vi "Wheel of Doom Controller.vi"(8 "error in":errorcluster) -> ()   [LabVIEW 2019]
doc: "This VI executes continuously carrying out the current operation and responding to updates or new operations. It will often contain the timing or control code that is difficult to place directly in TeleOp. This VI generally opens all sensors and motors and isolates the rest of the robot code from knowing how the operations are carried out."
uses:
  <vilib>/Rock Robotics/WPI/Framework/Completion Status.ctl
  Wheel of Doom Setpoints.ctl
  Wheel of Doom Operations.ctl
  <vilib>/Rock Robotics/WPI/ThirdParty/REV Robotics/SPARK MAX/Typedef/Spark MAX Motor Type.ctl
  <vilib>/Rock Robotics/WPI/MotorControl/WPI_MotorControlDeviceRef.ctl
  <vilib>/Rock Robotics/WPI/MotorControl/WPI_MotorControlType.ctl
  <vilib>/Rock Robotics/SystemInterfaces/DIO/FPGA_DIOPWMChannel.ctl
  <vilib>/Rock Robotics/WPI/PWM/WPI_PWMDeadband.ctl
  <vilib>/Rock Robotics/SystemInterfaces/DIO/FPGA_DIOChannel.ctl
  <vilib>/Rock Robotics/WPI/DigitalInput/WPI_DigitalInputDevRef.ctl
  <vilib>/Rock Robotics/WPI/ThirdParty/REV Robotics/Color SensorV3/Typedef/Color Sensor V3 DevRef.ctl
  <vilib>/Rock Robotics/WPI/I2C/WPI_I2CDevRef.ctl
  <vilib>/Rock Robotics/SystemInterfaces/i2clib/i2c_bus.ctl
  <vilib>/Rock Robotics/WPI/Interrupt/WPI_InterruptRef.ctl
  <vilib>/Rock Robotics/SystemInterfaces/Interrupt/FPGA_InterruptIndex.ctl
  Wheel of Doom Slot State.ctl
  <vilib>/Rock Robotics/WPI/ThirdParty/REV Robotics/Color SensorV3/Typedef/Color Sensor V3 ProximityRate.ctl
  <vilib>/Rock Robotics/WPI/ThirdParty/REV Robotics/Color SensorV3/Typedef/Color Sensor V3 ProxResolution.ctl
  <vilib>/Rock Robotics/WPI/Counter/WPI_CounterDevRef.ctl
  <vilib>/Rock Robotics/SystemInterfaces/Counter/FPGA_CounterCtrSystemIndex.ctl
  <vilib>/Rock Robotics/WPI/ThirdParty/REV Robotics/SPARK MAX/Typedef/Spark MAX Status Frames.ctl
  <vilib>/Rock Robotics/WPI/ThirdParty/REV Robotics/SPARK MAX/Typedef/Spark MAX Control Type.ctl
  <vilib>/Rock Robotics/WPI/Counter/WPI_CounterDigitalInputToDigitalSource.vi
  <vilib>/Rock Robotics/SystemInterfaces/CounterEncoderSourceConvertion/FPGA_CounterEncoderSourceConvertionLVSourceTypeToFPGAType.vi
  <vilib>/Rock Robotics/WPI/Interrupt/WPI_InterruptCache.vi
  <vilib>/Rock Robotics/SystemInterfaces/Interrupt/FPGA_InterruptWriteConfiguration.vi
  Wheel of Doom State.vi
  Wheel of Doom Internal Global.vi
  <vilib>/Rock Robotics/SystemInterfaces/Interrupt/FPGA_WaitOnInterrupt.vi
  <vilib>/Rock Robotics/WPI/Utilities/WPI_UtilitiesTimebaseConstants.vi
  <vilib>/Rock Robotics/SystemInterfaces/Interrupt/FPGA_InterruptReadTimestamp.vi
  <vilib>/ptbypt/NI_PtbyPt.lvlib
panel:
  in  "Auto-Karen Speed":dbl=0.19
  in  "Reverse Time":u32=600
  out "Current Trip":bool
  in  "Intake Mode Current Trigger":dbl=15.0
  in  "Intake Mode Speed":dbl=0.19
  out "Shoot All Complete":bool=TRUE
  in  "Shoot All Time (ms)":u32=3000
  in  "Wheel of Doom Shot Voltage":dbl=4.4
  out "Current Slot":u32=4
  out "State":cluster{"Valid":bool, "State":bool}[](array[cluster])=[{"Valid"=FALSE, "State"=FALSE}, {"Valid"=FALSE, "State"=FALSE}, {"Valid"=FALSE, "State"=FALSE}, {"Valid"=FALSE, "State"=FALSE}, {"Valid"=TRUE, "State"=FALSE}, {"Valid"=FALSE, "State"=FALSE}]
  out "Sensor Data":cluster{"Prox Threshold":u16, dbl}(graph)={"Prox Threshold"=14, 341.057373046875}
  in  "Prox Threshold":u16=30
  in  "Sensor Sample Start Pos":dbl
  in  "Sensor Sample End Pos":dbl
  in  "Interactive Values":T1
  out "Current\nCmd":string="Started at  19:17:32.261\n: Immediate,  S 0.0, D 0.000000"
  in  "Buttons":cluster{"Execute Cmd":bool, "Abort Cmd":bool}
  out "Command Timing":cluster{"Start Time (ms)":u32, "Iterations":i32}={"Start Time (ms)"=527443, "Iterations"=0}
  out "Status":T3
  # "Interactive Command: You may fill in the settings for a command\nand schedule it with the Execute button. You can observe and abort\nany command while fine tuning the code for the controller."
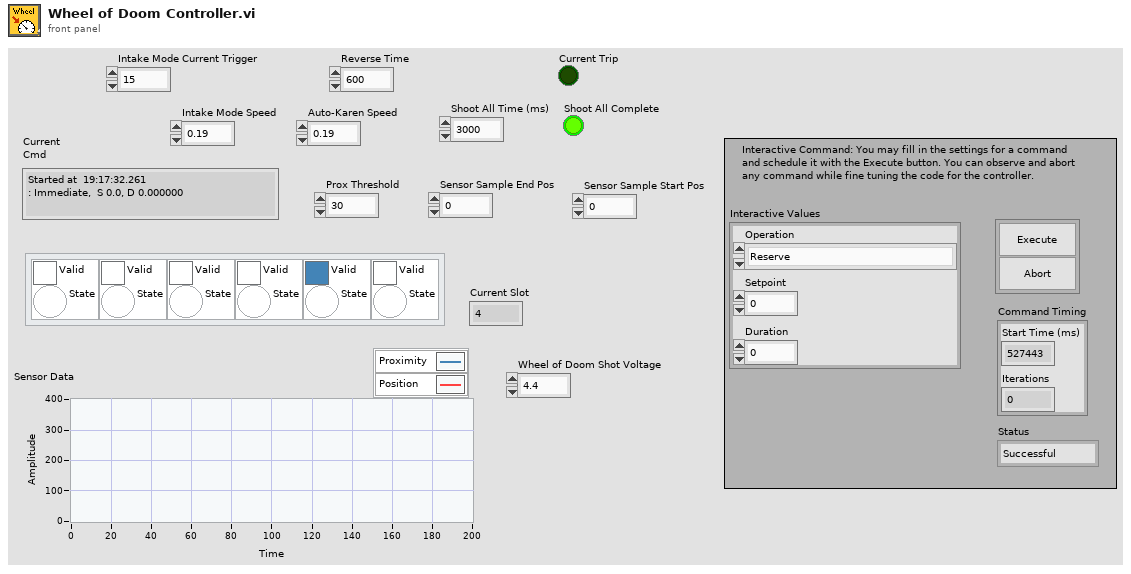
[diagram p1: front panel]
types:
  T1 = typedef "Wheel of Doom Setpoints.ctl" = cluster{"Operation":T2, "Setpoint":dbl, "Duration":dbl}
  T2 = typedef "Wheel of Doom Operations.ctl" = enum16{"Reserve", "Read Current", "Immediate", "Intake Mode", "Stop on Empty", "Shoot All", "Shoot One", "Stop", "Auto Karen"}
  T3 = typedef "Completion Status.ctl" = enum16{"Successful", "Aborted", "Incomplete"}
  T4 = typedef "Spark MAX Status Frames.ctl" = enum16{"Status 0", "Status 1", "Status 2", "Status 3"}
  T5 = typedef "Wheel of Doom Slot State.ctl" = cluster{"Slot Seen?":bool, "Ball Present":bool}
  T6 = typedef "WPI_MotorControlDeviceRef.ctl" = cluster{"DeviceStatus":errorcluster, "Type":T7, "PWM":cluster{"PWM Channel":T8, "DeadBand":T9}, "CAN":cluster{"Device Number":u8, "SetOutput VI Ref":variant, "GetOutput VI Ref":variant, "Enable VI Ref":variant, "Disable VI Ref":variant, "Data":variant}, "Invert":bool, "DIO PWM":cluster{"PWM \"Enable\" Channel":T8, "DIOChannel":T10, "PWM Rate":dbl}}
  T7 = typedef "WPI_MotorControlType.ctl" = enum16{"PWM", "CAN", "DIO PWM"}
  T8 = typedef "FPGA_DIOPWMChannel.ctl" = enum8{"PWM 0", "PWM 1", "PWM 2", "PWM 3", "PWM 4", "PWM 5", "PWM 6", "PWM 7", "PWM 8", "PWM 9", "PWM MXP 0", "PWM MXP 1", "PWM MXP 2", "PWM MXP 3", "PWM MXP 4", "PWM MXP 5", "PWM MXP 6", "PWM MXP 7", "PWM MXP 8", "PWM MXP 9", "Invalid"}
  T9 = typedef "WPI_PWMDeadband.ctl" = cluster{"Name":string, "maxPositivePwm":i32, "minPositivePwm":i32, "centerPwm":i32, "maxNegativePwm":i32, "minNegativePwm":i32, "angularRange":u16}
  T10 = typedef "FPGA_DIOChannel.ctl" = enum8{"DIO 0", "DIO 1", "DIO 2", "DIO 3", "DIO 4", "DIO 5", "DIO 6", "DIO 7", "DIO 8", "DIO 9", "DIO MXP 0", "DIO MXP 1", "DIO MXP 2", "DIO MXP 3", "DIO MXP 4", "DIO MXP 5", "DIO MXP 6", "DIO MXP 7", "DIO MXP 8", "DIO MXP 9", "DIO MXP 10", "DIO MXP 11", "DIO MXP 12", "DIO MXP 13", "DIO MXP 14", "DIO MXP 15", "SPI Port CS1", "SPI Port CS2", "SPI Port CS3", "SPI Port MISO", "SPI Port MOSI", "Invalid"}
  T11 = typedef "WPI_CounterDevRef.ctl" = cluster{"DevStatus":errorcluster, "CntIndex":T12}
  T12 = typedef "FPGA_CounterCtrSystemIndex.ctl" = enum8{"Ctr 0", "Ctr 1", "Ctr 2", "Ctr 3", "Ctr 4", "Ctr 5", "Ctr 6", "Ctr 7", "Invalid"}
  T13 = typedef "i2c_bus.ctl" = enum16{"I2C On-Board", "I2C MXP", "Invalid"}
  T14 = typedef "Color Sensor V3 ProxResolution.ctl" = enum8{"8bit", "9bit", "10bit", "11bit"}
  T15 = typedef "Color Sensor V3 ProximityRate.ctl" = enum16{"6ms", "12ms", "25ms", "50ms", "100ms", "200ms", "400ms"}
  T16 = typedef "WPI_DigitalInputDevRef.ctl" = cluster{"DevStatus":errorcluster, "DIO Channel":T10}
  T17 = typedef "Color Sensor V3 DevRef.ctl" = cluster{"I2CDevRef":T18}
  T18 = typedef "WPI_I2CDevRef.ctl" = cluster{"DevStatus":errorcluster, "Device Address":u8, "Handle":i32, "I2C Bus":T13}
  T19 = typedef "WPI_InterruptRef.ctl" = cluster{"DevStatus":errorcluster, "InterruptIndex":T20}
  T20 = typedef "FPGA_InterruptIndex.ctl" = enum8{"0", "1", "2", "3", "4", "5", "6", "7", "Invalid"}
  T21 = cluster{"Motor":T6, "Mag Switch":T16, "Prox Sensor":T17, "Interrupt":T19, "Slot States":T5[]}
  T22 = typedef "Spark MAX Motor Type.ctl" = enum16{"Brushed", "Brushless"}
  T23 = typedef "FPGA_CounterEncoderSourceConvertionLVSourceType.ctl" = cluster{"DevStatus":errorcluster, "AnalogTriggerMode?":bool, "DigitalMode":cluster{"DIO Channel":T24}, "AnalogTriggerMode":cluster{"AnalogTriggerIndex":T25, "OutputType":T26}}
  T24 = typedef "FPGA_DIODigitalSourceChannel.ctl" = enum8{"DIO 0", "DIO 1", "DIO 2", "DIO 3", "DIO 4", "DIO 5", "DIO 6", "DIO 7", "DIO 8", "DIO 9", "DIO MXP 0", "DIO MXP 1", "DIO MXP 2", "DIO MXP 3", "DIO MXP 4", "DIO MXP 5", "DIO MXP 6", "DIO MXP 7", "DIO MXP 8", "DIO MXP 9", "DIO MXP 10", "DIO MXP 11", "DIO MXP 12", "DIO MXP 13", "DIO MXP 14", "DIO MXP 15", "SPI Port CS1", "SPI Port CS2", "SPI Port CS3", "SPI Port MISO", "SPI Port MOSI", "Disabled"}
  T25 = typedef "FPGA_AnalogTriggerIndex.ctl" = enum8{"Trig 0", "Trig 1", "Trig 2", "Trig 3", "Trig 4", "Trig 5", "Trig 6", "Trig 7", "Invalid"}
  T26 = typedef "FPGA_AnalogTriggerOutType.ctl" = enum16{"InWindow", "TriggerState", "Rising", "Falling"}
  T27 = typedef "Command Status Info.ctl" = cluster{"Name":string, "Status":T3, "notifier out":T28}
  T28 = typedef "Completion Notifier.ctl" = refnum<notifier>
  T29 = cluster{"Current Command":T1, "Command Timing":cluster{"Start Time (ms)":u32, "Iterations":i32}, "Command Arguments":cluster{"Command Info":T27, "Description":string, "Default Command":T1, "queue out":refnum<queue>, "Subsystem Name":string}}
  T30 = typedef "Spark MAX Control Type.ctl" = enum16{"Percent VBus", "Voltage", "Velocity", "Position", "Smart Motion", "Current", "Smart Velocity"}
  T31 = cluster{"Proximity":u16, "Normalized Sensor Positon":dbl}
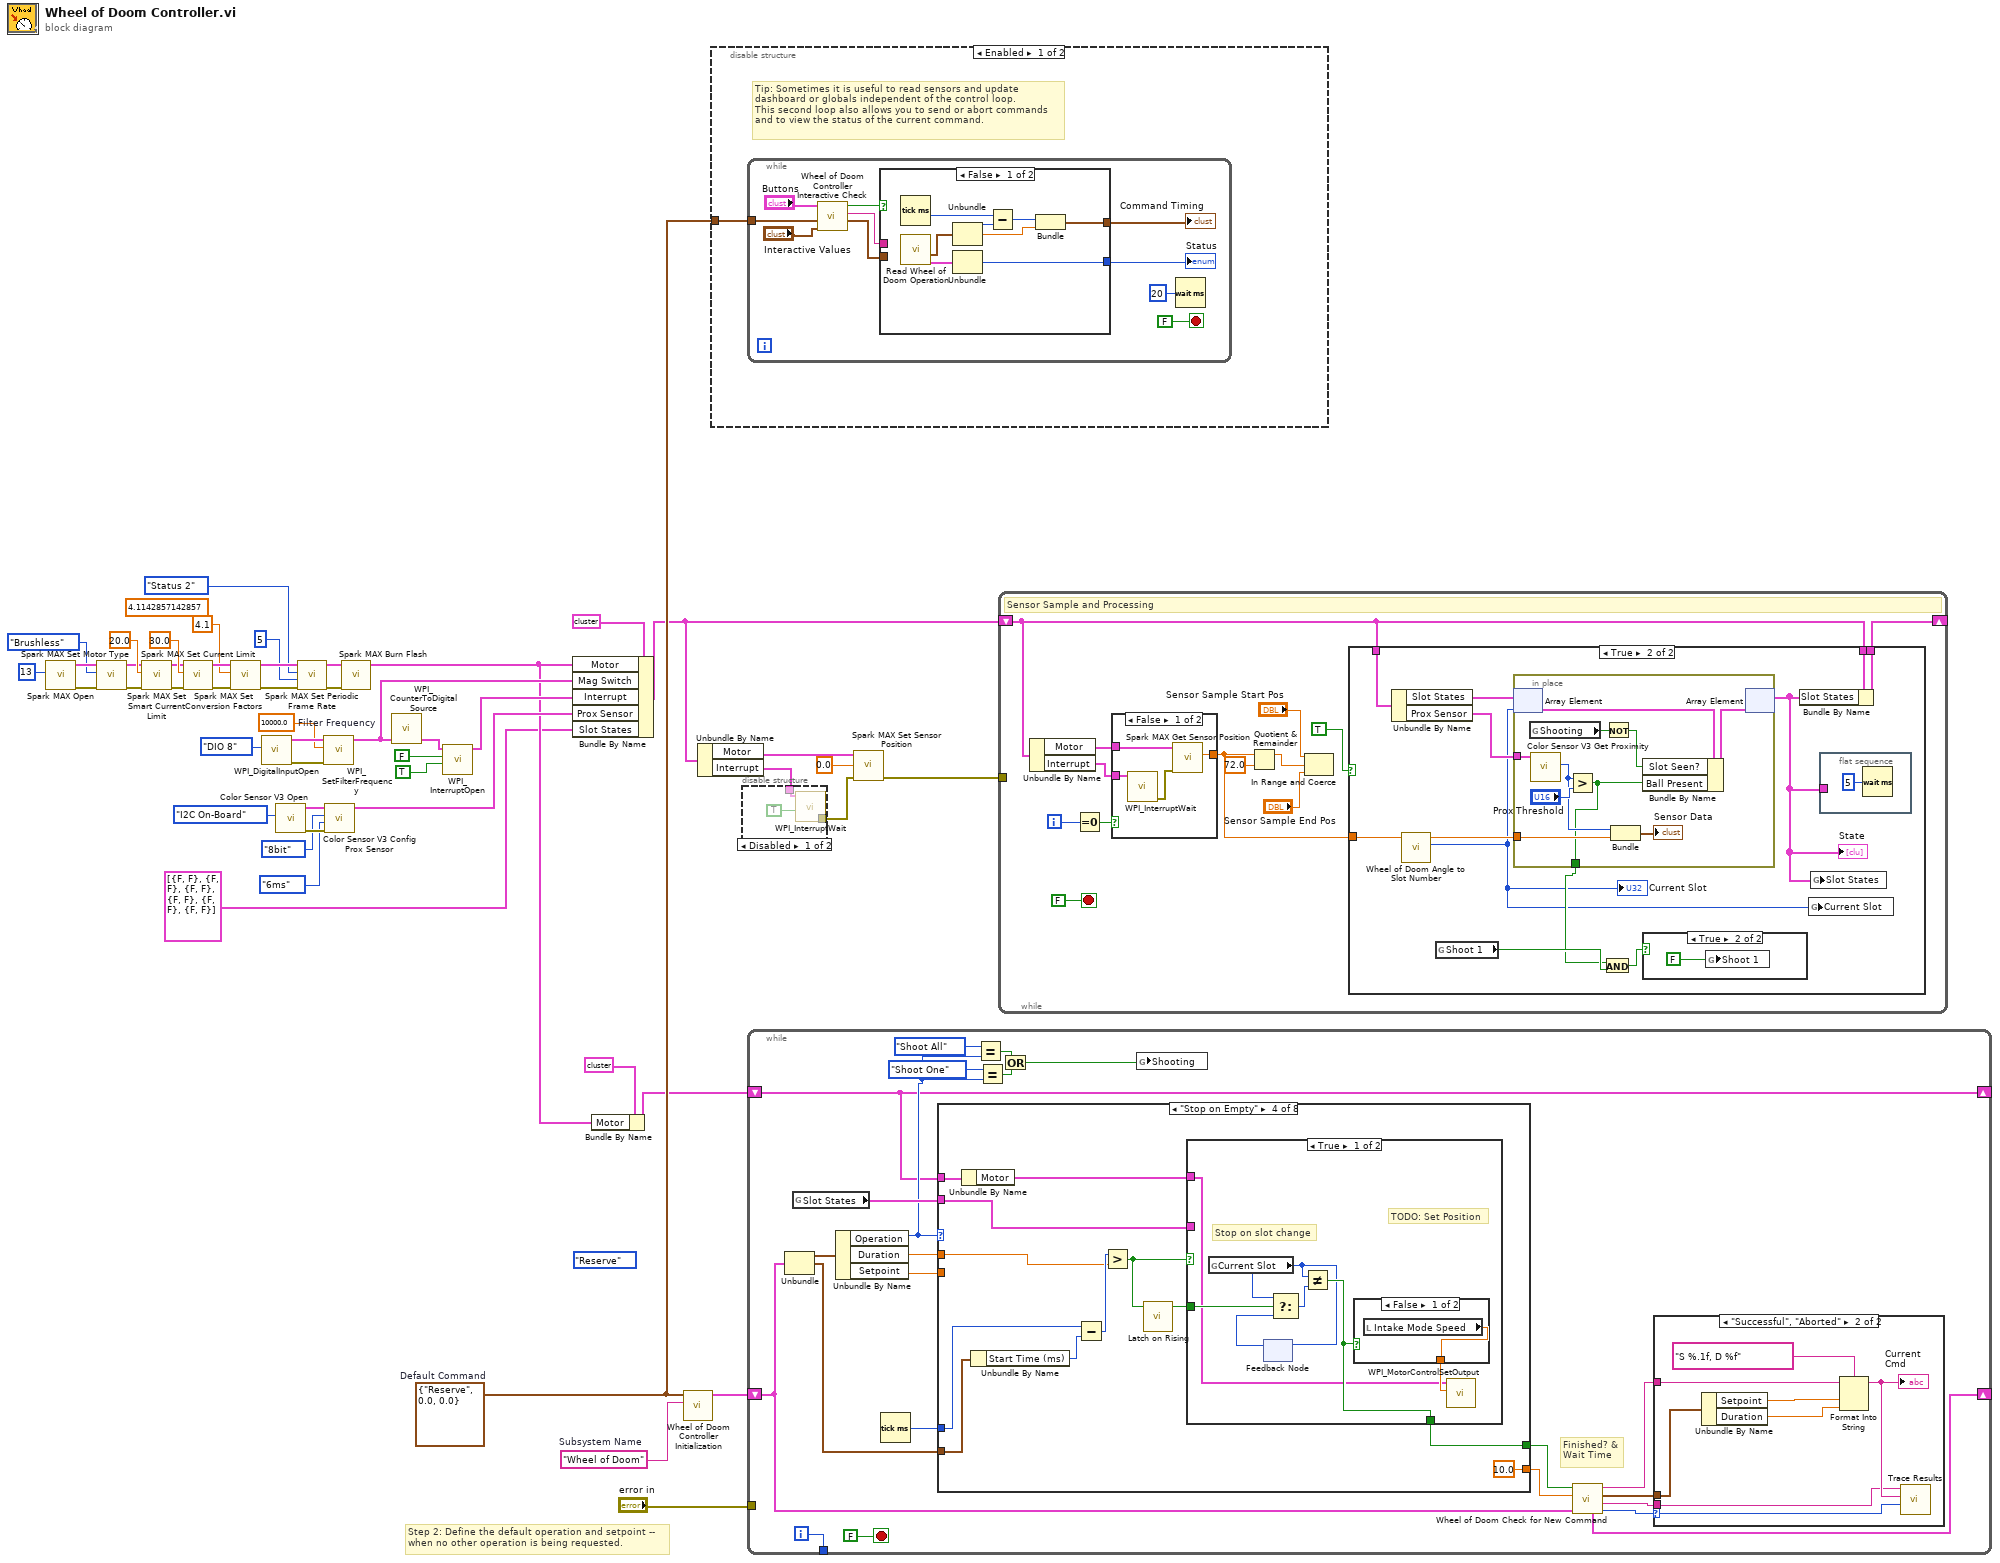
[diagram p0: block diagram]
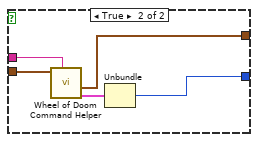
[diagram p2: hidden frame]
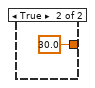
[diagram p5: hidden frame]
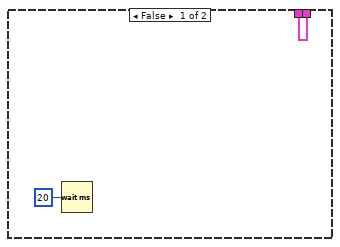
[diagram p6: hidden frame]
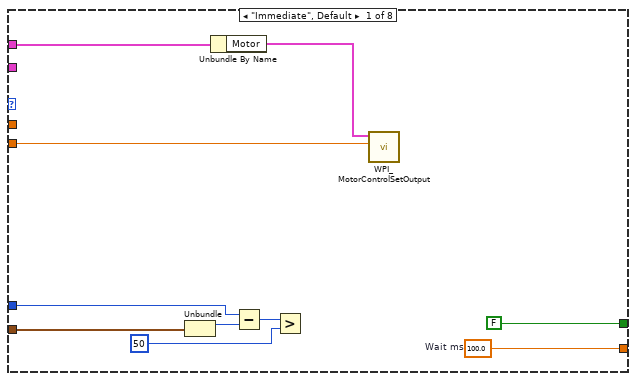
[diagram p9: hidden frame]
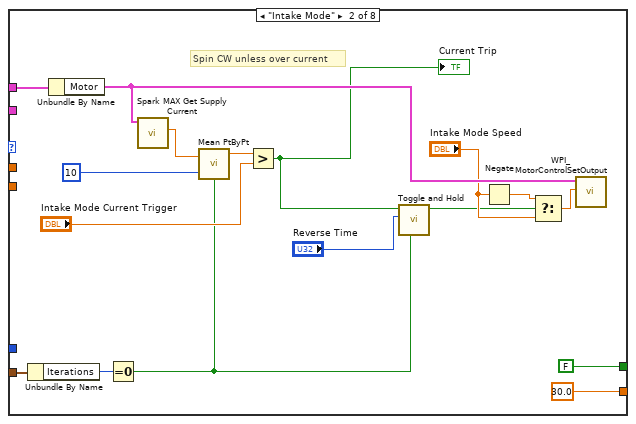
[diagram p10: hidden frame]
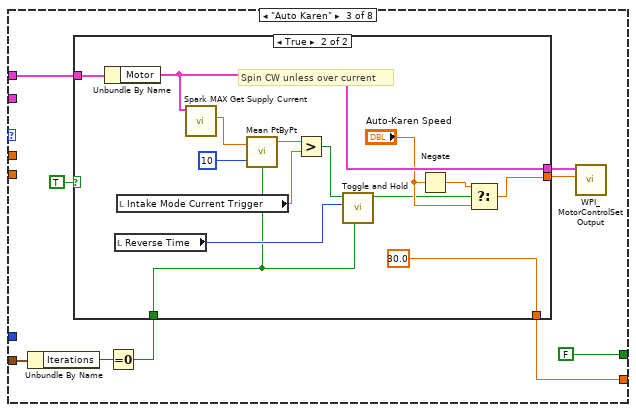
[diagram p11: hidden frame]
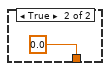
[diagram p13: hidden frame]
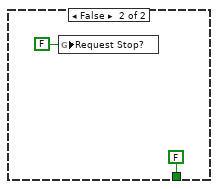
[diagram p14: hidden frame]
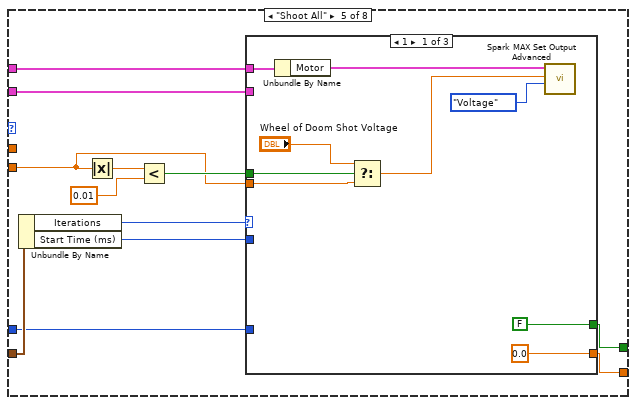
[diagram p15: hidden frame]
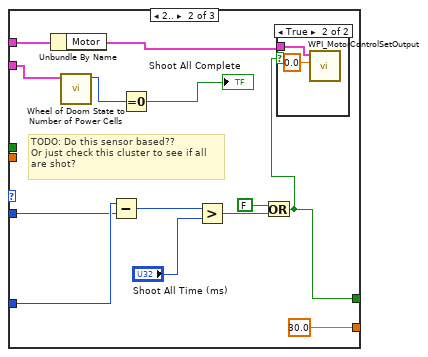
[diagram p16: hidden frame]
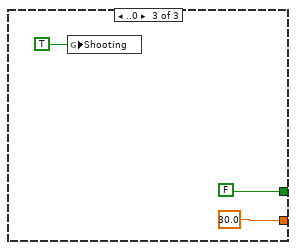
[diagram p18: hidden frame]
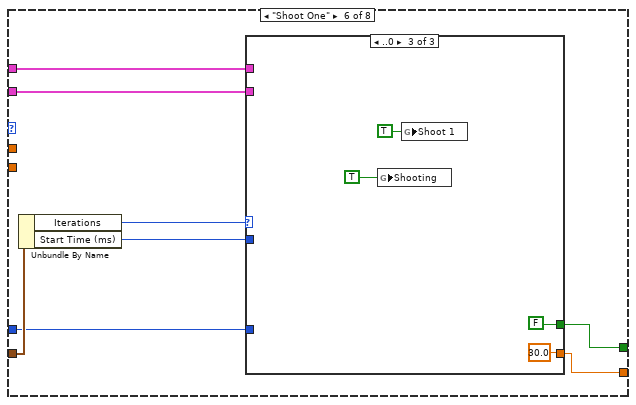
[diagram p19: hidden frame]
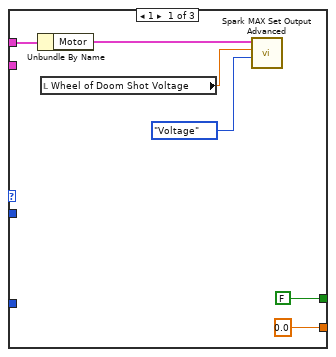
[diagram p20: hidden frame]
diagram:
  (unwired) 4.1142857142857 ("Position Factor (1)")
  (unwired) Wheel_of_Doom_Operations."Reserve" ("Operation")
  w31 = 10000.0  # Filter Frequency
  w46 = T1 {"Operation"=enum."Reserve", "Setpoint"=0.0, "Duration"=0.0}  # Default Command
  w47 = "Wheel of Doom"  # Subsystem Name
  # "Step 2: Define the default operation and setpoint --\nwhen no other operation is being requested."
  n1 = call <vilib>:"Spark MAX Open.vi"("Device Number"=u8 13) -> ("error out"=w42:errorcluster, "MotorControlDeviceRef"=w38:T6)  [unwired: 9 in]
  n2 = call <vilib>:"Spark MAX Set Motor Type.vi"("error in (no error)"=w42, "Motor Type"=Spark_MAX_Motor_Type."Brushless", "MotorControlDevRef"=w38) -> ("error out"=w39:errorcluster, "MotorControlDeviceRef"=w37:T6)  [unwired: 7 in]
  n3 = call <vilib>:"Spark MAX Set Smart Current Limit.vi"("error in (no error)"=w39, "Primay Current Limit (80A)"=20.0, "MotorControlDeviceRef in"=w37) -> ("error out"=w40:errorcluster, "MotorControlDeviceRef out"=w41:T6)  [unwired: 7 in]
  n4 = call <vilib>:"Spark MAX Set Current Limit.vi"("error in (no error)"=w40, "Current Limit A (100)"=sgl 30.0, "MotorControlDeviceRef in"=w41) -> ("error out"=w35:errorcluster, "MotorControlDeviceRef out"=w8:T6)  [unwired: 7 in]
  n5 = call <vilib>:"Spark MAX Set Conversion Factors.vi"("error in (no error)"=w35, "Position Factor (1)"=4.1, "MotorControlDeviceRef in"=w8) -> ("error out"=w9:errorcluster, "MotorControlDeviceRef out"=w6:T6)  [unwired: 7 in]
  n6 = call <vilib>:"WPI_DigitalInputOpen.vi"("DIO Channel"=FPGA_DIOChannel."DIO 8") -> ("error out"=w32:errorcluster, "DigitalInputDevRef"=w34:T16)  [unwired: 9 in]
  n7 = call <vilib>:"Color Sensor V3 Open.vi"("I2C Bus"=i2c_bus."I2C On-Board") -> ("error out"=w30:errorcluster, "ColorSensorDevRef"=w29:T17)  [unwired: 9 in]
  n8 = call <vilib>:"Spark MAX Set Periodic Frame Rate.vi"("error in"=w9, "Frame rate (ms)"=u16 5, "Frame"=Spark_MAX_Status_Frames."Status 2", "MotorControlDeviceRef"=w6) -> ("error out"=w7:errorcluster, "MotorControlDeviceRef"=w5:T6)  [unwired: 6 in]
  n9 = call <vilib>:"WPI_SetFilterFrequency.vi"("error in (no error)"=w32, "Filter Frequency"=w31, "DigitalInputDevRef"=w34) -> ("DigitalInputDevRef"=w25:T16)  [unwired: 7 in, 1 out]
  n10 = call <vilib>:"Color Sensor V3 Config Prox Sensor.vi"("error in (no error)"=w30, "ProximitySensorMeasurementRate"=Color_Sensor_V3_ProximityRate."6ms", "ProximitySensorResolution"=Color_Sensor_V3_ProxResolution."8bit", "ColorSensorDevRef"=w29) -> ("ColorSensorDevRef out"=w17:T17)  [unwired: 6 in, 1 out]
  n11 = call <vilib>:"Spark MAX Burn Flash.vi"("error in"=w7, "MotorControlDeviceRef"=w5) -> ("MotorControlDeviceRef"=w11:T6)  [unwired: 8 in, 1 out]
  n12 = call-poly <vilib>:"WPI_CounterToDigitalSource.vi"("DigitalInputDevRef"=w25) -> ("Digital Source"=w24:T23)  [unwired: 6 in]
  n13 = call <vilib>:"WPI_InterruptOpen.vi"("Falling Edge"=TRUE, "Rising Edge"=FALSE, "Source"=w24) -> ("InterruptRef"=w16:T19)  [unwired: 7 in, 1 out]
  n14 = Bundle By Name(cluster=T21 {"Motor"={"DeviceStatus"={"status"=FALSE, "code"=0, "source"=""}, "Type"=enum."PWM", "PWM"={"PWM Channel"=enum."Invalid", "DeadBand"={"Name"="", "maxPositivePwm"=0, "minPositivePwm"=0, "centerPwm"=0, "maxNegativePwm"=0, "minNegativePwm"=0, "angularRange"=0}}, "CAN"={"Device Number"=0, "SetOutput VI Ref"=variant(refnum<vi> refnum), "GetOutput VI Ref"=variant(refnum<vi> refnum), "Enable VI Ref"=variant(refnum<vi> refnum), "Disable VI Ref"=variant(refnum<vi> refnum), "Data"=variant}, "Invert"=FALSE, "DIO PWM"={"PWM \"Enable\" Channel"=enum."Invalid", "DIOChannel"=enum."Invalid", "PWM Rate"=0.0}}, "Mag Switch"={"DevStatus"={"status"=FALSE, "code"=0, "source"=""}, "DIO Channel"=enum."DIO 1"}, "Prox Sensor"={"I2CDevRef"={"DevStatus"={"status"=FALSE, "code"=0, "source"=""}, "Device Address"=0, "Handle"=0, "I2C Bus"=enum."Invalid"}}, "Interrupt"={"DevStatus"={"status"=FALSE, "code"=0, "source"=""}, "InterruptIndex"=enum."Invalid"}, "Slot States"=[{"Slot Seen?"=FALSE, "Ball Present"=FALSE}, {"Slot Seen?"=FALSE, "Ball Present"=FALSE}, {"Slot Seen?"=FALSE, "Ball Present"=FALSE}, {"Slot Seen?"=FALSE, "Ball Present"=FALSE}, {"Slot Seen?"=FALSE, "Ball Present"=FALSE}]}, "Motor"=w11, "Mag Switch"=w25, "Interrupt"=w16, "Prox Sensor"=w17, "Slot States"=T5[] [{"Slot Seen?"=FALSE, "Ball Present"=FALSE}, {"Slot Seen?"=FALSE, "Ball Present"=FALSE}, {"Slot Seen?"=FALSE, "Ball Present"=FALSE}, {"Slot Seen?"=FALSE, "Ball Present"=FALSE}, {"Slot Seen?"=FALSE, "Ball Present"=FALSE}, {"Slot Seen?"=FALSE, "Ball Present"=FALSE}]) -> (w2:T21)
  n15 = Bundle By Name(cluster=cluster{"Motor":T6, "Ball Detect2":T11} {"Motor"={"DeviceStatus"={"status"=FALSE, "code"=0, "source"=""}, "Type"=enum."PWM", "PWM"={"PWM Channel"=enum."Invalid", "DeadBand"={"Name"="", "maxPositivePwm"=0, "minPositivePwm"=0, "centerPwm"=0, "maxNegativePwm"=0, "minNegativePwm"=0, "angularRange"=0}}, "CAN"={"Device Number"=0, "SetOutput VI Ref"=variant(refnum<vi> refnum), "GetOutput VI Ref"=variant(refnum<vi> refnum), "Enable VI Ref"=variant(refnum<vi> refnum), "Disable VI Ref"=variant(refnum<vi> refnum), "Data"=variant}, "Invert"=FALSE, "DIO PWM"={"PWM \"Enable\" Channel"=enum."Invalid", "DIOChannel"=enum."Invalid", "PWM Rate"=0.0}}, "Ball Detect2"={"DevStatus"={"status"=FALSE, "code"=0, "source"=""}, "CntIndex"=enum."Ctr 0"}}, "Motor"=w11) -> (w12:cluster{"Motor":T6, "Ball Detect2":T11})
  n16 = call "Wheel of Doom Controller Initialization.vi"("Subsystem Name"=w47, "Default Command"=w46) -> ("Current Command"=w48:T29)  [unwired: 9 in]
  n17 = Unbundle By Name(w2) -> ("Motor"=w20:T6, "Interrupt"=w14:T19)
  n18 = disable-structure shown="Enabled" {
    disable-tunnel: w46 -> [w50 _]
    frame Enabled {
      # "Tip: Sometimes it is useful to read sensors and update\ndashboard or globals independent of the control loop.\nThis second loop also allows you to send or abort commands\nand to view the status of the current command."
      n19 = while {
        tunnel: w50 -> [w57]
        stop <- FALSE stop-if-true
        n20 = call "Wheel of Doom Controller Interactive Check.vi"("Interactive Command in"="Interactive Values", "Default Command"=w57, "Buttons"="Buttons") -> ("Interactive Command out"=w54:T1, "Trace String"=w55:string, "Schedule"=w56:bool)  [unwired: 6 in]
        n21 = case shown="False" w56 {
          tunnel: [w68 w73] -> w53
          tunnel: w54 -> [_ w71]
          tunnel: [w64 w69] -> w52
          tunnel: w55 -> [_ w72]
          frame False {
            n22 = Tick Count (ms)() -> (millisecond timer value=w63:u32)
            n23 = call "Read Wheel of Doom Operation.vi"() -> ("Command Info"=w61:T27, "SubSystem Data"=w62:T1)  [unwired: 9 in, 1 out]
            n24 = Unbundle(w62) -> ("Operation"=w67:T2, "Setpoint"=w65:dbl)  [unwired: 1 out]
            n25 = Unbundle(w61) -> ("Status"=w68:T3)  [unwired: 2 out]
            n26 = Subtract(x=w63, y=w67) -> (x-y=w66:u32)
            n27 = Bundle(w66, "Setpoint"=w65) -> (w64:cluster{u32, "Setpoint":dbl})  [unwired: 1 in]
          }
          frame True {
            n28 = call "Wheel of Doom Command Helper.vi"("Description"=w72, "SubSystem Data"=w71) -> ("Command Info Out"=w70:T27, "Command Timing"=w69:cluster{"Start Time (ms)":u32, "Iterations":i32})  [unwired: 7 in, 1 out]
            n29 = Unbundle(w70) -> ("Status"=w73:T3)  [unwired: 2 out]
          }
        }
        "Status" <- w53
        "Command Timing" <- w52
        n30 = Wait (ms)(milliseconds to wait=u32 20) -> ()  [unwired: 1 out]
      }
    }
    frame Disabled {
    }
  }
  n31 = disable-structure shown="Disabled" {
    disable-tunnel: [w75 _] -> w21
    disable-tunnel: w14 -> [w74 _]
    frame Disabled {
      n32 = call <vilib>:"WPI_InterruptWait.vi"("Ignore Previous Interrupts"=TRUE, "InterruptRef"=w74) -> ("error out"=w75:errorcluster)  [unwired: 5 in, 4 out]
    }
    frame Enabled {
    }
  }
  n33 = while {
    shift-right: [w93] -> _
    shift-left: w48 -> [w86]
    tunnel: [w98] -> _
    tunnel: "error in" -> [_]
    shift-right: [w77] -> _
    shift-left: w12 -> [w77]
    i -> [w98]
    stop <- FALSE stop-if-true
    # "Finished? &\nWait Time"
    n34 = Unbundle(w86) -> ("Current Command"=w97:T1, "Command Timing"=w95:cluster{"Start Time (ms)":u32, "Iterations":i32})  [unwired: 1 out]
    n35 = global read "Wheel of Doom State.vi" "Slot States"() -> (w84:T5[])
    n36 = Unbundle By Name(w97) -> ("Operation"=w80:T2, "Duration"=w85:dbl, "Setpoint"=w94:dbl)
    n37 = Tick Count (ms)() -> (millisecond timer value=w96:u32)
    n38 = case shown="\"Stop on Empty\"" w80 {
      tunnel: [w117 30.0 ("Infinite") w142 10.0 ("Infinite") w189 w224 w246 0.0 ("Infinite")] -> w91
      tunnel: [FALSE ("ignore previous (F)") FALSE ("ignore previous (F)") FALSE ("ignore previous (F)") w165 w188 w223 FALSE ("ignore previous (F)") TRUE ("ignore previous (F)")] -> w92
      tunnel: w95 -> [w113 w130 w139 w166 w192 w227 _ _]
      tunnel: w85 -> [_ _ _ w160 _ _ _ _]
      tunnel: w96 -> [w112 _ _ w162 w187 w222 _ _]
      tunnel: w94 -> [w109 _ _ _ w181 _ _ _]
      tunnel: w84 -> [_ _ _ w167 w185 w220 _ _]
      tunnel: w77 -> [w111 w132 w141 w169 w190 w225 _ w249]
      frame "Immediate", Default {
        w117 = 100.0  # Wait ms
        n39 = Unbundle(w113) -> ("Start Time (ms)"=w116:u32)  [unwired: 1 out]
        n40 = Unbundle By Name(w111) -> ("Motor"=w110:T6)
        n41 = Subtract(x=w112, y=w116) -> (x-y=w115:u32)
        n42 = Greater?(x=w115, y=u8 50 ("Left Motor")) -> ()  [unwired: 1 out]
        n43 = call <vilib>:"WPI_MotorControlSetOutput.vi"("Output"=w109, "MotorControlDevRef"=w110) -> ()  [unwired: 7 in, 3 out]
      }
      frame "Intake Mode" {
        # "Spin CW unless over current"
        n44 = Unbundle By Name(w130) -> ("Iterations"=w129:i32)
        n45 = Unbundle By Name(w132) -> ("Motor"=w131:T6)
        n46 = Equal To 0?(x=w129) -> (x = 0?=w120:bool)
        n47 = call <vilib>:"Spark MAX Get Supply Current.vi"("MotorControlDevRef in"=w131) -> ("Current"=w127:dbl)  [unwired: 7 in, 3 out]
        n48 = call <vilib>:"Mean PtByPt.vi"("x"=w127, "sample length"=10, "initialize"=w120) -> ("mean"=w126:dbl)  [unwired: 1 in, 1 out]
        n49 = Greater?(x=w126, y="Intake Mode Current Trigger") -> (0:w118:bool)
        "Current Trip" <- w118
        n50 = call "Toggle and Hold.vi"("Reset? (F)"=w120, "Hold Time (ms)"="Reverse Time", "Trigger"=w118) -> ("Toggled?"=w119:bool)  [unwired: 7 in, 1 out]
        n51 = Negate(x="Intake Mode Speed") -> (-x=w123:dbl)
        n52 = Select(t=w123, s=w119, f="Intake Mode Speed") -> (s? t:f=w124:dbl)
        n53 = call <vilib>:"WPI_MotorControlSetOutput.vi"("Output"=w124, "MotorControlDevRef"=w131) -> ()  [unwired: 7 in, 3 out]
      }
      frame "Auto Karen" {
        n54 = Unbundle By Name(w139) -> ("Iterations"=w138:i32)
        n55 = Equal To 0?(x=w138) -> (x = 0?=w137:bool)
        n56 = case shown="True" TRUE {
          tunnel: [_ 30.0 ("Infinite")] -> w142
          tunnel: w141 -> [_ w156]
          tunnel: [_ w155] -> w140
          tunnel: w137 -> [_ w146]
          tunnel: [_ w144] -> w136
          frame False {
          }
          frame True {
            # "Spin CW unless over current"
            n57 = Unbundle By Name(w156) -> ("Motor"=w155:T6)
            n58 = local read "Reverse Time"() -> (w147:u32)
            n59 = local read "Intake Mode Current Trigger"() -> (w148:dbl)
            n60 = call <vilib>:"Spark MAX Get Supply Current.vi"("MotorControlDevRef in"=w155) -> ("Current"=w153:dbl)  [unwired: 7 in, 3 out]
            n61 = call <vilib>:"Mean PtByPt.vi"("x"=w153, "sample length"=10, "initialize"=w146) -> ("mean"=w152:dbl)  [unwired: 1 in, 1 out]
            n62 = Greater?(x=w152, y=w148) -> (0:w145:bool)
            n63 = call "Toggle and Hold.vi"("Reset? (F)"=w146, "Hold Time (ms)"=w147, "Trigger"=w145) -> ("Toggled?"=w149:bool)  [unwired: 7 in, 1 out]
            n64 = Negate(x="Auto-Karen Speed") -> (-x=w151:dbl)
            n65 = Select(t=w151, s=w149, f="Auto-Karen Speed") -> (s? t:f=w144:dbl)
          }
        }
        n66 = call <vilib>:"WPI_MotorControlSetOutput.vi"("Output"=w136, "MotorControlDevRef"=w140) -> ()  [unwired: 7 in, 3 out]
      }
      frame "Stop on Empty" {
        n67 = Unbundle By Name(w169) -> ("Motor"=w168:T6)
        n68 = Unbundle By Name(w166) -> ("Start Time (ms)"=w163:u32)
        n69 = Subtract(x=w162, y=w163) -> (x-y=w161:u32)
        n70 = Greater?(x=w161, y=w160) -> (0:w159:bool)
        n71 = call <vilib>:"Latch on Rising.vi"("Boolean in"=w159) -> ("Boolean out"=w158:bool)  [unwired: 4 in]
        n72 = case shown="True" w159 {
          tunnel: w168 -> [w170 _]
          tunnel: w167 -> [_ _]
          tunnel: [w176 FALSE] -> w165
          tunnel: w158 -> [w172 _]
          frame True {
            # "Stop on slot change"
            # "TODO: Set Position"
            n73 = global read "Wheel of Doom State.vi" "Current Slot"() -> (w174:u32)
            n74 = feedback-in #1(w174) -> ()
            n75 = feedback #1() -> (w175:u32)  [unwired: 1 in]
            n76 = Select(t=w174, s=w172, f=w175) -> (s? t:f=w173:u32)
            n77 = Not Equal?(x=w174, y=w173) -> (x != y?=w176:bool)
            n78 = case shown="False" w176 {
              tunnel: [w177 0.0 ("Output")] -> w171
              frame False {
                n79 = local read "Intake Mode Speed"() -> (w177:dbl)
              }
              frame True {
              }
            }
            n80 = call <vilib>:"WPI_MotorControlSetOutput.vi"("Output"=w171, "MotorControlDevRef"=w170) -> ()  [unwired: 7 in, 3 out]
          }
          frame False {
            n81 = global write "Wheel of Doom State.vi" "Request Stop?"(FALSE ("Request Stop?")) -> ()
          }
        }
      }
      frame "Shoot All" {
        n82 = Unbundle By Name(w192) -> ("Iterations"=w191:i32, "Start Time (ms)"=w186:u32)
        n83 = Absolute Value(x=w181) -> (abs(x)=w184:dbl)
        n84 = Less?(x=w184, y=0.01) -> (x < y?=w182:bool)
        n85 = case shown="1" w191 {
          tunnel: w190 -> [w201 w207 _]
          tunnel: [0.0 30.0 30.0] -> w189
          tunnel: [FALSE w208 FALSE] -> w188
          tunnel: w187 -> [_ w214 _]
          tunnel: w186 -> [_ w213 _]
          tunnel: w185 -> [_ w206 _]
          tunnel: w182 -> [w196 _ _]
          tunnel: w181 -> [w193 _ _]
          frame 1 {
            n86 = Unbundle By Name(w201) -> ("Motor"=w200:T6)
            n87 = Select(t="Wheel of Doom Shot Voltage", s=w196, f=w193) -> (s? t:f=w194:dbl)
            n88 = call <vilib>:"Spark MAX Set Output Advanced.vi"("Control Mode"=Spark_MAX_Control_Type."Voltage", "Setpoint"=w194, "MotorControlDevRef"=w200) -> ()  [unwired: 7 in, 2 out]
          }
          frame 2.. {
            # "TODO: Do this sensor based??\nOr just check this cluster to see if all are shot?"
            n89 = Unbundle By Name(w207) -> ("Motor"=w203:T6)
            n90 = call "Wheel of Doom State to Number of Power Cells.vi"("Slot States"=w206) -> ("Numeric"=w205:i32)  [unwired: 10 in]
            n91 = Subtract(x=w214, y=w213) -> (x-y=w212:u32)
            n92 = Equal To 0?(x=w205) -> (x = 0?=→"Shoot All Complete":bool)
            n93 = Greater?(x=w212, y="Shoot All Time (ms)") -> (0:w209:bool)
            n94 = Or(x=FALSE, y=w209) -> (x .or. y?=w208:bool)
            n95 = case shown="True" w208 {
              tunnel: w203 -> [_ w216]
              frame False {
              }
              frame True {
                n96 = call <vilib>:"WPI_MotorControlSetOutput.vi"("Output"=0.0, "MotorControlDevRef"=w216) -> ()  [unwired: 7 in, 3 out]
              }
            }
          }
          frame ..0 {
            n97 = global write "Wheel of Doom Internal Global.vi" "Shooting"(TRUE ("Shooting All")) -> ()
          }
        }
      }
      frame "Shoot One" {
        n98 = Unbundle By Name(w227) -> ("Iterations"=w226:i32, "Start Time (ms)"=w221:u32)
        n99 = case shown="..0" w226 {
          tunnel: w225 -> [w233 w236 _]
          tunnel: [0.0 30.0 30.0] -> w224
          tunnel: [FALSE w234 FALSE] -> w223
          tunnel: w222 -> [_ _ _]
          tunnel: w221 -> [_ _ _]
          tunnel: w220 -> [_ _ _]
          frame 1 {
            n100 = Unbundle By Name(w233) -> ("Motor"=w232:T6)
            n101 = local read "Wheel of Doom Shot Voltage"() -> (w228:dbl)
            n102 = call <vilib>:"Spark MAX Set Output Advanced.vi"("Control Mode"=Spark_MAX_Control_Type."Voltage", "Setpoint"=w228, "MotorControlDevRef"=w232) -> ()  [unwired: 7 in, 2 out]
          }
          frame 2.. {
            n103 = global read "Wheel of Doom State.vi" "Shoot 1"() -> (w237:bool)
            n104 = Unbundle By Name(w236) -> ("Motor"=w235:T6)
            n105 = Not(x=w237) -> (.not. x?=w234:bool)
            n106 = case shown="True" w234 {
              tunnel: w235 -> [_ w240]
              frame False {
              }
              frame True {
                n107 = call <vilib>:"WPI_MotorControlSetOutput.vi"("Output"=0.0, "MotorControlDevRef"=w240) -> ()  [unwired: 7 in, 3 out]
              }
            }
          }
          frame ..0 {
            n108 = global write "Wheel of Doom Internal Global.vi" "Shooting"(TRUE ("Shooting All")) -> ()
            n109 = global write "Wheel of Doom State.vi" "Shoot 1"(TRUE ("Shoot 1")) -> ()
          }
        }
      }
      frame "Reserve" {
        w246 = 10.0  # Infinite
        # "If loop needs to poll sensors or other\nvalues, use a timeout value. -1 waits for\nnext command to be sent."
      }
      frame "Stop" {
        n110 = Unbundle By Name(w249) -> ("Motor"=w248:T6)
        n111 = call <vilib>:"WPI_MotorControlSetOutput.vi"("Output"=0.0, "MotorControlDevRef"=w248) -> ()  [unwired: 7 in, 3 out]
      }
    }
    n112 = Equal?(x=Wheel_of_Doom_Operations."Shoot All", y=w80) -> (x = y?=w83:bool)
    n113 = Equal?(x=Wheel_of_Doom_Operations."Shoot One", y=w80) -> (x = y?=w82:bool)
    n114 = Or(x=w83, y=w82) -> (x .or. y?=w81:bool)
    n115 = global write "Wheel of Doom Internal Global.vi" "Shooting"(w81) -> ()
    n116 = call "Wheel of Doom Check for New Command.vi"("Current Command"=w86, "Wait time (ms)"=w91, "Finished?"=w92) -> ("Completion"=w87:T3, "Subsystem Name"=w88:string, "Current Command"=w89:T1, "Initial Trace String"=w90:string, "NextCommand"=w93:T29)  [unwired: 4 in]
    n117 = case shown="\"Successful\", \"Aborted\"" w87 {
      selector: w87 -> [_ w107]
      tunnel: w90 -> [_ w103]
      tunnel: w89 -> [_ w104]
      tunnel: w88 -> [_ w100]
      frame "Incomplete", Default {
        # "Continuing current command"
      }
      frame "Successful", "Aborted" {
        # "Report and setup for next command"
        n118 = Unbundle By Name(w104) -> ("Setpoint"=w106:dbl, "Duration"=w101:dbl)
        n119 = Format Into String(format string="S %.1f, D %f", initial string=w103, w106, w101) -> (resulting string=w102:string)  [unwired: 1 in, 1 out]
        "Current\nCmd" <- w102
        n120 = call <vilib>:"Trace Results.vi"("Status of previous command"=w107, "Description"=w102, "Subsystem"=w100) -> ()  [unwired: 9 in]
      }
    }
  }
  n121 = call <vilib>:"Spark MAX Set Sensor Position.vi"("error in"=w21, "Position"=0.0, "MotorControlDeviceRef"=w20) -> ("error out"=w18:errorcluster)  [unwired: 7 in, 1 out]
  n122 = while {
    shift-right: [w261] -> _
    shift-left: w2 -> [w260]
    tunnel: w18 -> [_]
    i -> [w253]
    stop <- FALSE stop-if-true
    # "Sensor Sample and Processing"
    n123 = Unbundle By Name(w260) -> ("Motor"=w263:T6, "Interrupt"=w262:T19)
    n124 = Equal To 0?(x=w253) -> (x = 0?=w254:bool)
    n125 = case shown="False" w254 {
      tunnel: w263 -> [w268 _]
      tunnel: w262 -> [w267 _]
      tunnel: [w265 30.0 ("Sensor Position")] -> w256
      frame False {
        n126 = call <vilib>:"WPI_InterruptWait.vi"("InterruptRef"=w267) -> ("error out"=w266:errorcluster)  [unwired: 6 in, 4 out]
        n127 = call <vilib>:"Spark MAX Get Sensor Position.vi"("error in (no error)"=w266, "MotorControlDevRef in"=w268) -> ("Sensor Position"=w265:dbl)  [unwired: 6 in, 3 out]
      }
      frame True {
      }
    }
    n128 = Quotient & Remainder(x=w256, y=72.0) -> (x-y*floor(x/y)=w255:dbl)  [unwired: 1 out]
    n129 = In Range and Coerce(upper limit="Sensor Sample Start Pos", x=w255, lower limit="Sensor Sample End Pos") -> ()  [unwired: 2 out]
    n130 = case shown="True" TRUE {
      tunnel: w260 -> [_ w283]
      tunnel: w256 -> [_ w282]
      tunnel: w260 -> [w270 w281]
      tunnel: [w270 w280] -> w261
      frame False {
        n131 = Wait (ms)(milliseconds to wait=u32 20) -> ()  [unwired: 1 out]
      }
      frame True {
        n132 = Unbundle By Name(w283) -> ("Slot States"=w279:T5[], "Prox Sensor"=w278:T17)
        n133 = call "Wheel of Doom Angle to Slot Number.vi"("Sensor Position"=w282) -> ("Slot Number"=w272:u32, "Normalized Sensor Positon"=w277:dbl)  [unwired: 9 in]
        "Current Slot" <- w272
        n134 = global read "Wheel of Doom State.vi" "Shoot 1"() -> (w274:bool)
        n135 = in-place {
          in-place-border: w278 -> [w295]
          in-place-border: w277 -> [w290]
          in-place-border: [w286] -> w273
          n136 = in-place-array #2(w279, w272) -> (w294:T5)
          n137 = global read "Wheel of Doom Internal Global.vi" "Shooting"() -> (w288:bool)
          n138 = call <vilib>:"Color Sensor V3 Get Proximity.vi"("ColorSensorDevRef"=w295) -> ("Proximity"=w287:u16)  [unwired: 8 in, 2 out]
          n139 = Greater?(x=w287, y="Prox Threshold") -> (0:w286:bool)
          n140 = Not(x=w288) -> (.not. x?=w289:bool)
          n141 = Bundle("Proximity"=w287, "Normalized Sensor Positon"=w290) -> (→"Sensor Data":T31)  [unwired: 1 in]
          n142 = Bundle By Name(cluster=w294, "Slot Seen?"=w289, "Ball Present"=w286) -> (w293:T5)
          n143 = in-place-array #2(w293) -> (w276:T5[])  [unwired: 1 out]
        }
        "State" <- w276
        n144 = And(x=w273, y=w274) -> (x .and. y?=w275:bool)
        n145 = case shown="True" w275 {
          frame False {
          }
          frame True {
            n146 = global write "Wheel of Doom State.vi" "Shoot 1"(FALSE ("Request Stop?")) -> ()
          }
        }
        n147 = Bundle By Name(cluster=w281, "Slot States"=w276) -> (w280:T21)
        n148 = global write "Wheel of Doom State.vi" "Current Slot"(w272) -> ()
        n149 = global write "Wheel of Doom State.vi" "Slot States"(w276) -> ()
        n150 = flat-sequence {
          tunnel: w276 -> [_]
          frame #0 {
            n151 = Wait (ms)(milliseconds to wait=u32 5) -> ()  [unwired: 1 out]
          }
        }
      }
    }
  }
